vi "Init.vi"(3 "Which Index":i32) -> (1 "Act_Delete One.lvclass":refnum<class "Act_Delete One.lvclass">)   [LabVIEW 2014, in "Act_Delete One.lvclass"]
uses:
  Act_Delete One.lvclass
  Act_Delete One.lvclass/Act_Delete One.ctl
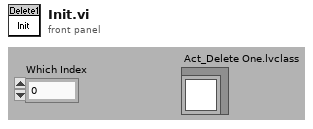
[diagram p1: front panel]
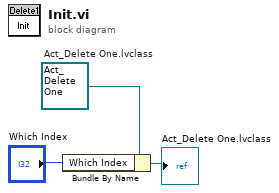
[diagram p0: block diagram]
diagram:
  w2 = refnum<class "Act_Delete One.lvclass"> refnum  # Act_Delete One.lvclass
  n1 = Bundle By Name(cluster=w2, "Which Index"="Which Index") -> (→"Act_Delete One.lvclass":refnum<class "Act_Delete One.lvclass">)
